vi "Enable New Unit.vi"(0 "Unit Abbreviations In":string[](array[string]), 5 "Units In":string[](array[string]), 7 "Abbreviation":string, 9 "ID":string caption="ID (usually max pt.)", 11 "Result":string, 12 "NewCalPts":dbl[](array[numeric]) caption="Suggested Calibration Setpoints", 13 "NewVerPts":dbl[](array[numeric]) caption="Suggested Verification Points") -> (4 "Unit Abbreviations Out":string[](array[string]), 6 "Units Out":string[](array[string]), 10 "Valid?":bool, 15 "Duplicate":bool)   [LabVIEW 2019]
panel:
  # "(5)"
  # "(10)"
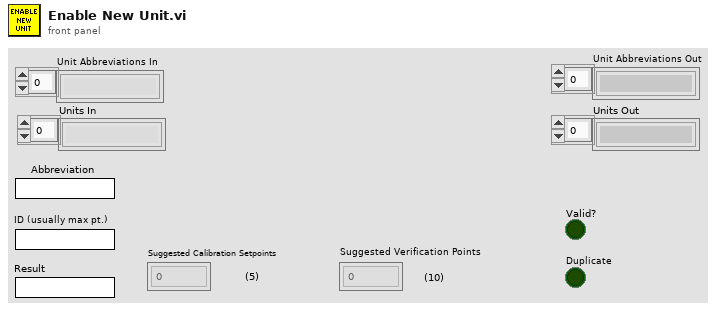
[diagram p1: front panel]
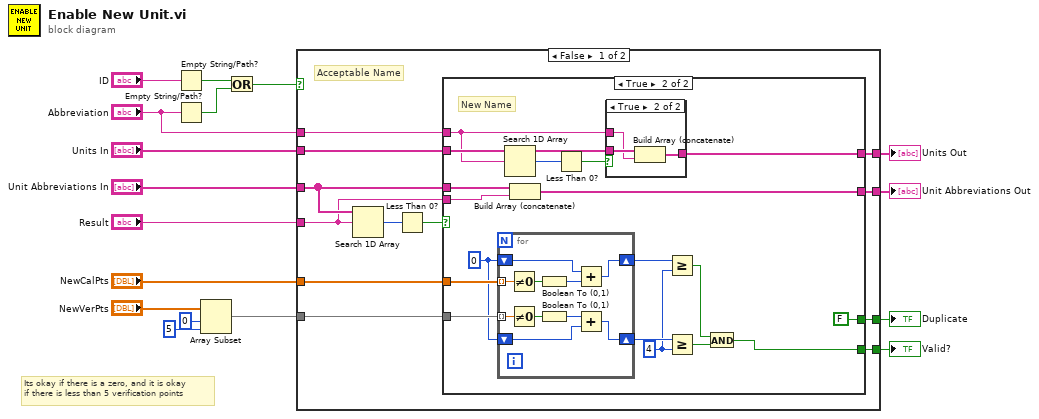
[diagram p0: block diagram]
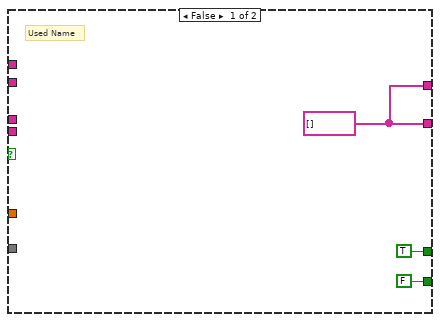
[diagram p2: hidden frame]
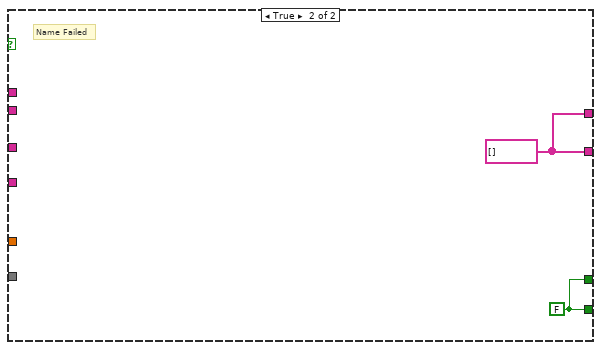
[diagram p4: hidden frame]
diagram:
  # "Its okay if there is a zero, and it is okay\nif there is less than 5 verification points"
  n1 = Empty String/Path?(string/path="ID") -> (empty?=w7:bool)
  n2 = Empty String/Path?(string/path="Abbreviation") -> (empty?=w8:bool)
  n3 = Array Subset(array="NewVerPts", index=0, length=5) -> (w1:dbl[])
  n4 = Or(x=w7, y=w8) -> (x .or. y?=w16:bool)
  n5 = case shown="False" w16 {
    tunnel: [w27 w66] -> w15
    tunnel: "Abbreviation" -> [w22 _]
    tunnel: "Unit Abbreviations In" -> [w25 _]
    tunnel: "Result" -> [w24 _]
    tunnel: [w26 w66] -> w11
    tunnel: [w23 w65] -> w10
    tunnel: "Units In" -> [w21 _]
    tunnel: [w20 w65] -> w6
    tunnel: "NewCalPts" -> [w19 _]
    tunnel: w1 -> [w18 _]
    frame False {
      # "Acceptable Name"
      n6 = Search 1D Array(1D array=w25, element=w24) -> (index of element=w29:i32)  [unwired: 1 in]
      n7 = Less Than 0?(x=w29) -> (x < 0?=w28:bool)
      n8 = case shown="True" w28 {
        tunnel: [FALSE w33] -> w27
        tunnel: [TRUE FALSE] -> w26
        tunnel: w25 -> [_ w48]
        tunnel: w24 -> [_ w49]
        tunnel: [w30 w47] -> w23
        tunnel: w22 -> [_ w43]
        tunnel: w21 -> [_ w44]
        tunnel: [w30 w42] -> w20
        tunnel: w19 -> [_ w41]
        tunnel: w18 -> [_ w40]
        frame False {
          w30 = string[] []
          # "Used Name"
        }
        frame True {
          w36 = i16 4 ("y")
          w39 = i16 0
          # "New Name"
          n9 = for {
            tunnel: w41 -> [w59] mode=indexing
            tunnel: w40 -> [w60] mode=indexing
            shift-right: [w53] -> w37
            shift-left: w39 -> [w51]
            shift-right: [w54] -> w38
            shift-left: w39 -> [w52]
            n10 = Not Equal To 0?(x=w59) -> (x != 0?=w58:bool)
            n11 = Not Equal To 0?(x=w60) -> (x != 0?=w57:bool)
            n12 = Boolean To (0,1)(Boolean=w58) -> (0, 1=w55:i16)
            n13 = Boolean To (0,1)(Boolean=w57) -> (0, 1=w56:i16)
            n14 = Add(x=w52, y=w55) -> (x+y=w54:i16)
            n15 = Add(x=w56, y=w51) -> (x+y=w53:i16)
          }
          n16 = Search 1D Array(1D array=w44, element=w43) -> (index of element=w46:i32)  [unwired: 1 in]
          n17 = Build Array (concatenate)(w48, w49) -> (w47:string[])
          n18 = Less Than 0?(x=w46) -> (x < 0?=w45:bool)
          n19 = case shown="True" w45 {
            tunnel: w44 -> [w61 w64]
            tunnel: w43 -> [_ w63]
            tunnel: [w61 w62] -> w42
            frame False {
            }
            frame True {
              n20 = Build Array (concatenate)(w64, w63) -> (w62:string[])
            }
          }
          n21 = Greater Or Equal?(x=w38, y=w36) -> (x >= y?=w35:bool)
          n22 = Greater Or Equal?(x=w37, y=w36) -> (x >= y?=w34:bool)
          n23 = And(x=w35, y=w34) -> (x .and. y?=w33:bool)
        }
      }
    }
    frame True {
      w65 = string[] []
      w66 = FALSE
      # "Name Failed"
    }
  }
  "Valid?" <- w15
  "Duplicate" <- w11
  "Unit Abbreviations Out" <- w10
  "Units Out" <- w6
